vi "trigonometric operations.vi"() -> ()   [LabVIEW 2017]
panel:
  out "tan(x)":dbl
  out "cos(x)":dbl
  out "sin(x)":dbl
  out "x*y":dbl
  in  "degree":dbl
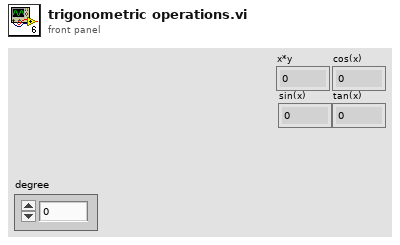
[diagram p1: front panel]
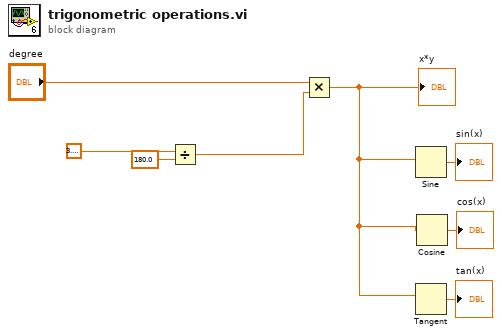
[diagram p0: block diagram]
diagram:
  n1 = Divide(x=3.141592653589793, y=180.0) -> (x/y=w5:dbl)
  n2 = Multiply(x="degree", y=w5) -> (x*y=w4:dbl)
  "x*y" <- w4
  n3 = Sine(x=w4) -> (sin(x)=→"sin(x)":dbl)
  n4 = Tangent(1:w4) -> (0:→"tan(x)":dbl)
  n5 = Cosine(x=w4) -> (cos(x)=→"cos(x)":dbl)
